vi "RichToFlatcif_manager_ClockStatusArray.vi"(5 "OutputClusterType":T1, 11 "InputCluster":T5) -> (3 "OutputCluster":T1)   [LabVIEW 2021, in "CIF_Launcher_server.lvlib"]
uses:
  CIF_Launcher_server.lvlib
  cif_manager_ClockStatusArray.ctl
  cif_manager_ClockStatus.ctl
  cif_manager_ClockConversion.ctl
  cif_manager_TimePair.ctl
  cif_manager_ClockStatusArray_Flat.ctl
  cif_manager_ClockStatus_Flat.ctl
  cif_manager_ClockConversion_Flat.ctl
  cif_manager_TimePair_Flat.ctl
  RichToFlatcif_manager_ClockConversion.vi
  RichToFlatcif_manager_TimePair.vi
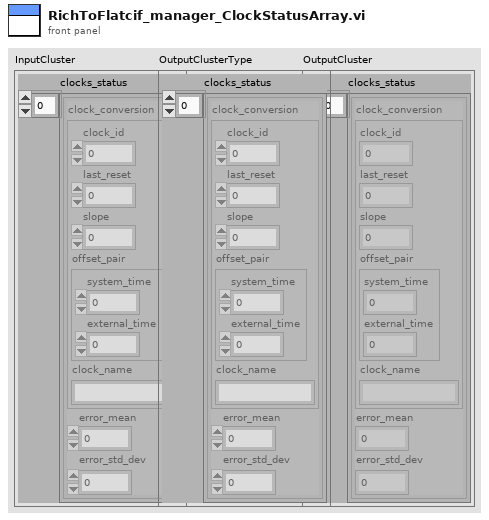
[diagram p1: front panel]
types:
  T1 = typedef "CIF_Launcher_server.lvlib/cif_manager_ClockStatusArray_Flat.ctl" = cluster{"clocks_status":T2[]}
  T2 = typedef "CIF_Launcher_server.lvlib/cif_manager_ClockStatus_Flat.ctl" = cluster{"clock_conversion":T3, "error_mean":i64, "error_std_dev":i64}
  T3 = typedef "CIF_Launcher_server.lvlib/cif_manager_ClockConversion_Flat.ctl" = cluster{"clock_id":u32, "last_reset":i64, "slope":dbl, "offset_pair":T4, "clock_name":string}
  T4 = typedef "CIF_Launcher_server.lvlib/cif_manager_TimePair_Flat.ctl" = cluster{"system_time":i64, "external_time":i64}
  T5 = typedef "CIF_Launcher_server.lvlib/cif_manager_ClockStatusArray.ctl" = cluster{"clocks_status":T6[]}
  T6 = typedef "CIF_Launcher_server.lvlib/cif_manager_ClockStatus.ctl" = cluster{"clock_conversion":T7, "error_mean":i64, "error_std_dev":i64}
  T7 = typedef "CIF_Launcher_server.lvlib/cif_manager_ClockConversion.ctl" = cluster{"clock_id":u32, "last_reset":i64, "slope":dbl, "offset_pair":T8, "clock_name":string}
  T8 = typedef "CIF_Launcher_server.lvlib/cif_manager_TimePair.ctl" = cluster{"system_time":i64, "external_time":i64}
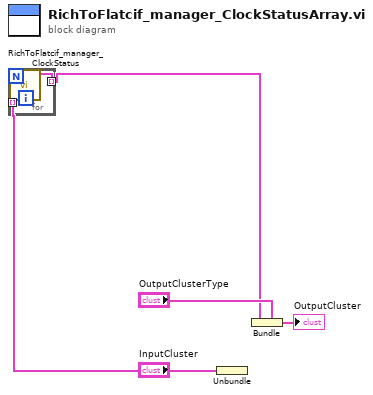
[diagram p0: block diagram]
diagram:
  n1 = Unbundle "Unbundle"("InputCluster") -> ("clocks_status"=w2:T6[])
  n2 = for {
    tunnel: w2 -> [w7] mode=indexing
    tunnel: [w6] -> w1 mode=indexing
    n3 = call "RichToFlatcif_manager_ClockStatus.vi"("InputCluster"=w7) -> ("OutputCluster"=w6:T2)  [unwired: 10 in]
  }
  n4 = Bundle "Bundle"(cluster="OutputClusterType", "clocks_status"=w1) -> (→"OutputCluster":T1)
